vi "SelectTubel.vi"(8 "error in (no error)":errorcluster, 10 "Unique Object Identifier":string, 11 "DataHandler in":refnum<class "DataHandler.lvclass">) -> (0 "error out":errorcluster, 1 "ControlParameterArray":string[](array[string]), 2 "Control Parameter":T1, 3 "DataHandler out":refnum<class "DataHandler.lvclass">)   [LabVIEW 2017, in "DataHandler.lvclass"]
uses:
  DataHandler.lvclass
  DataHandler.lvclass/DataHandler.ctl
  <vilib>/drjdpowell/SQLite Library/SQL Statement/SQL Statement.lvclass/SQL Statement.ctl
  <vilib>/drjdpowell/SQLite Library/SQL Statement/Column I64.vi
  <vilib>/drjdpowell/SQLite Library/SQL Statement/Column DBL.vi
  <vilib>/drjdpowell/SQLite Library/SQL Statement/Step.vi
  <vilib>/drjdpowell/SQLite Library/SQL Statement/Column Type.vi
  <vilib>/drjdpowell/SQLite Library/SQL Statement/Error Message.vi
  <vilib>/drjdpowell/SQLite Library/SQL Statement/Column String.vi
  <vilib>/drjdpowell/SQLite Library/SQL Statement/SQL Statement.lvclass
  <vilib>/drjdpowell/SQLite Library/SQL Connection/Connection.lvclass
panel:
  # "Cunsumer, Produzer, Converter (CPC)"
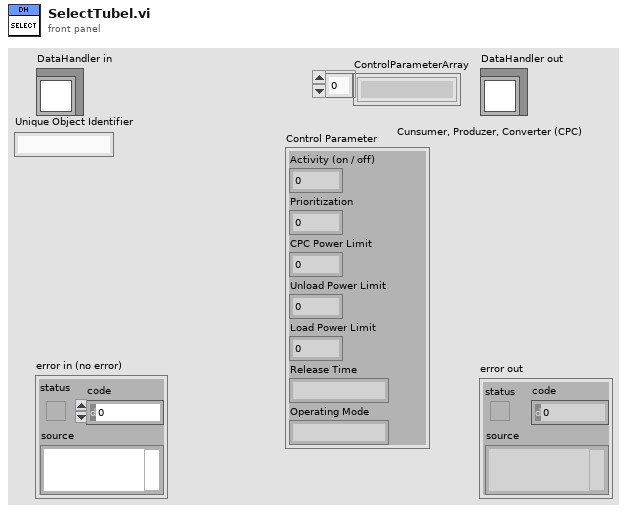
[diagram p1: front panel]
types:
  T1 = cluster{"Activity (on / off)":i64, "Prioritization":i64, "CPC Power Limit":dbl, "Unload Power Limit":dbl, "Load Power Limit":dbl, "Release Time":string, "Operating Mode":string}
  T2 = cluster{"Column:Get Column I64":i64, "Column:Get Column I64":i64, "Column:Get Column DBL":dbl, "Column:Get Column DBL":dbl, "Column:Get Column DBL":dbl, "Column:Get Column String":string, "Column:Get Column String":string}
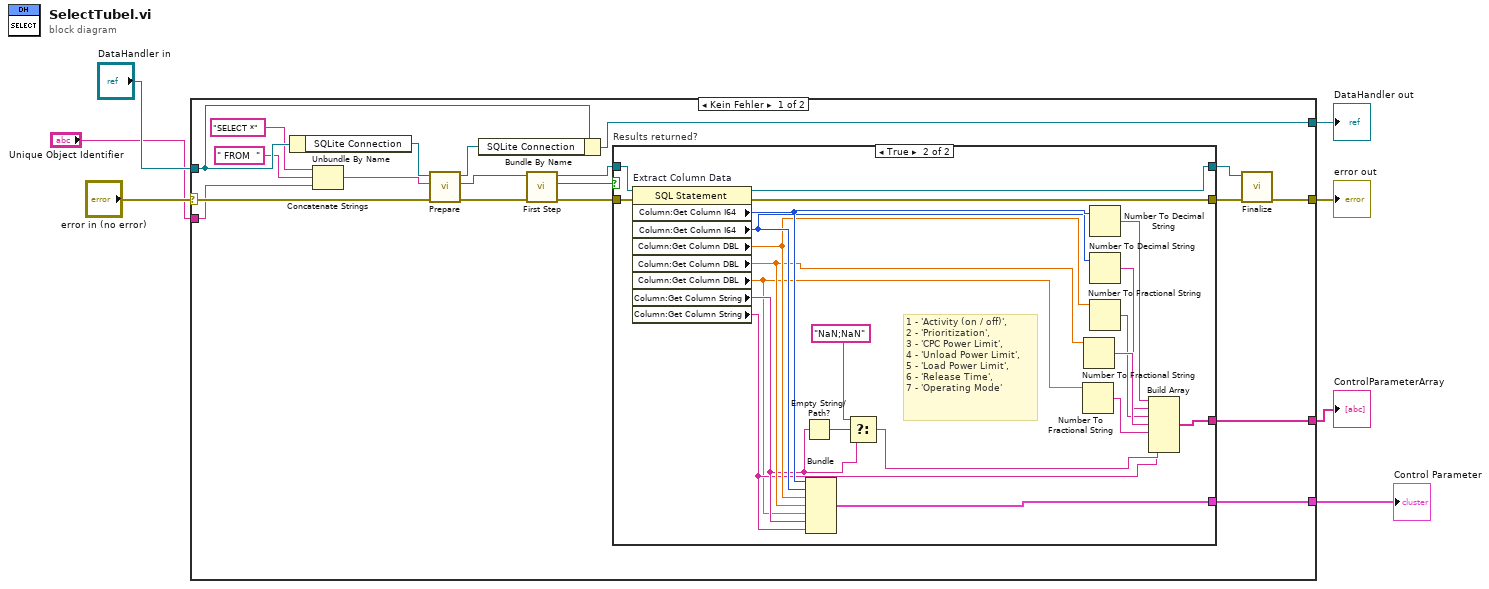
[diagram p0: block diagram]
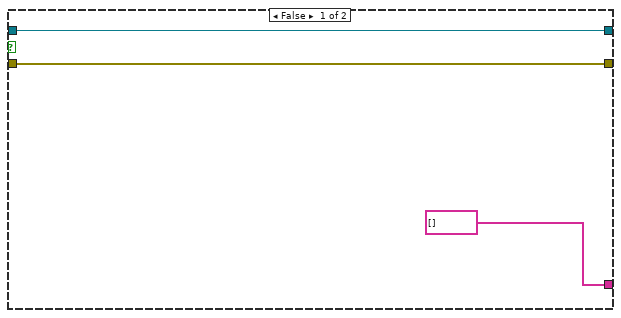
[diagram p2: hidden frame]
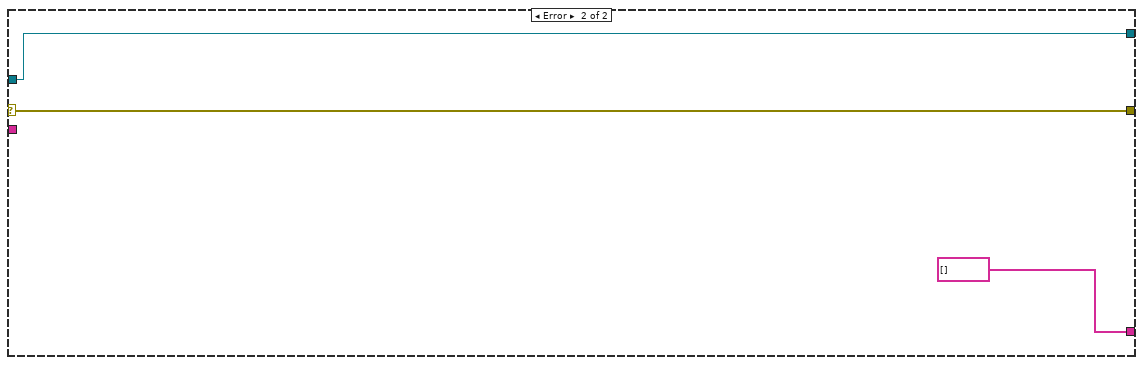
[diagram p3: hidden frame]
diagram:
  n1 = case shown="Kein Fehler" "error in (no error)" {
    selector: "error in (no error)" -> [w15 w53]
    tunnel: [w14 w53] -> w6
    tunnel: [w17 w52] -> w4
    tunnel: "DataHandler in" -> [w18 w52]
    tunnel: "Unique Object Identifier" -> [w12 _]
    tunnel: [w10 _] -> w2
    tunnel: [w8 string[] []] -> w1
    frame No Error {
      n2 = Unbundle By Name(w18) -> ("SQLite Connection"=w19:refnum<class "Connection.lvclass">)
      n3 = Concatenate Strings("SELECT *" ("string"), " FROM  " ("string"), w12) -> (w11:string)
      n4 = call <vilib>:"Prepare.vi"("error in (no error)"=w15, "SQL"=w11, "SQLite Connection in"=w19) -> ("error out"=w20:errorcluster, "SQL Statement"=w21:refnum<class "SQL Statement.lvclass">, "SQLite Connection"=w16:refnum<class "Connection.lvclass">)  [unwired: 4 in, 2 out]
      n5 = Bundle By Name(cluster=w18, "SQLite Connection"=w16) -> (w17:refnum<class "DataHandler.lvclass">)
      n6 = call <vilib>:"First Step.vi"("error in (no error)"=w20, "SQL Statement in"=w21) -> ("error out"=w23:errorcluster, "Row returned"=w22:bool, "SQL Statement"=w24:refnum<class "SQL Statement.lvclass">)  [unwired: 7 in]
      n7 = case "Results returned?" shown="True" w22 {
        tunnel: [w29 w47] -> w25
        tunnel: [w28 w48] -> w26
        tunnel: w24 -> [w29 w50]
        tunnel: w23 -> [w28 w49]
        tunnel: [_ w46] -> w10
        tunnel: [string[] [] w37] -> w8
        frame False {
        }
        frame True {
          # "1 - 'Activity (on / off)', \n2 - 'Prioritization', \n3 - 'CPC Power Limit',  \n4 - 'Unload Power Limit',\n5 - 'Load Power Limit',\n6 - 'Release Time',\n7 - 'Operating Mode'"
          n8 = property on="Extract Column Data" class="SQL Statement"(reference=w50, error in=w49) -> (reference out=w47:refnum<class "SQL Statement.lvclass">, error out=w48:errorcluster, "Column:Get Column I64"=w45:i64, "Column:Get Column I64"=w44:i64, "Column:Get Column DBL"=w43:dbl, "Column:Get Column DBL"=w42:dbl, "Column:Get Column DBL"=w30:dbl, "Column:Get Column String"=w33:string, "Column:Get Column String"=w32:string)
          n9 = Empty String/Path?(string/path=w33) -> (empty?=w36:bool)
          n10 = Bundle("Column:Get Column I64"=w45, "Column:Get Column I64"=w44, "Column:Get Column DBL"=w43, "Column:Get Column DBL"=w42, "Column:Get Column DBL"=w30, "Column:Get Column String"=w33, "Column:Get Column String"=w32) -> (w46:T2)  [unwired: 1 in]
          n11 = Select(t="NaN;NaN", s=w36, f=w33) -> (s? t:f=w34:string)
          n12 = Number To Fractional String(number=w30) -> (F-format string=w31:string)  [unwired: 3 in]
          n13 = Number To Fractional String(number=w42) -> (F-format string=w41:string)  [unwired: 3 in]
          n14 = Number To Decimal String(number=w45) -> (decimal integer string=w38:string)  [unwired: 1 in]
          n15 = Number To Decimal String(number=w44) -> (decimal integer string=w39:string)  [unwired: 1 in]
          n16 = Number To Fractional String(number=w43) -> (F-format string=w40:string)  [unwired: 3 in]
          n17 = Build Array(w38, w39, w40, w41, w31, w34, w32) -> (w37:string[])
        }
      }
      n18 = call <vilib>:"Finalize.vi"("error in (no error)"=w26, "SQL Statement in"=w25) -> ("error out"=w14:errorcluster)  [unwired: 9 in]
    }
    frame Error {
    }
  }
  "error out" <- w6
  "DataHandler out" <- w4
  "Control Parameter" <- w2
  "ControlParameterArray" <- w1
